vi "Cockpit UDP Receive.vi"(8 "error in":errorcluster, 11 "connection ID":refnum<k16>) -> (0 "error out":errorcluster, 2 "read UDP array":sgl[](array[numeric]), 3 "connection ID out":refnum<k16>)   [LabVIEW 2016]
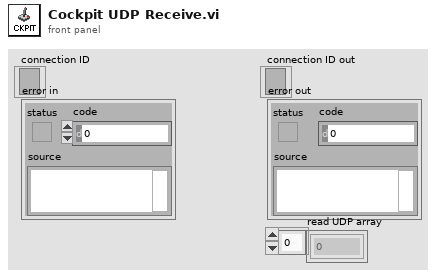
[diagram p1: front panel]
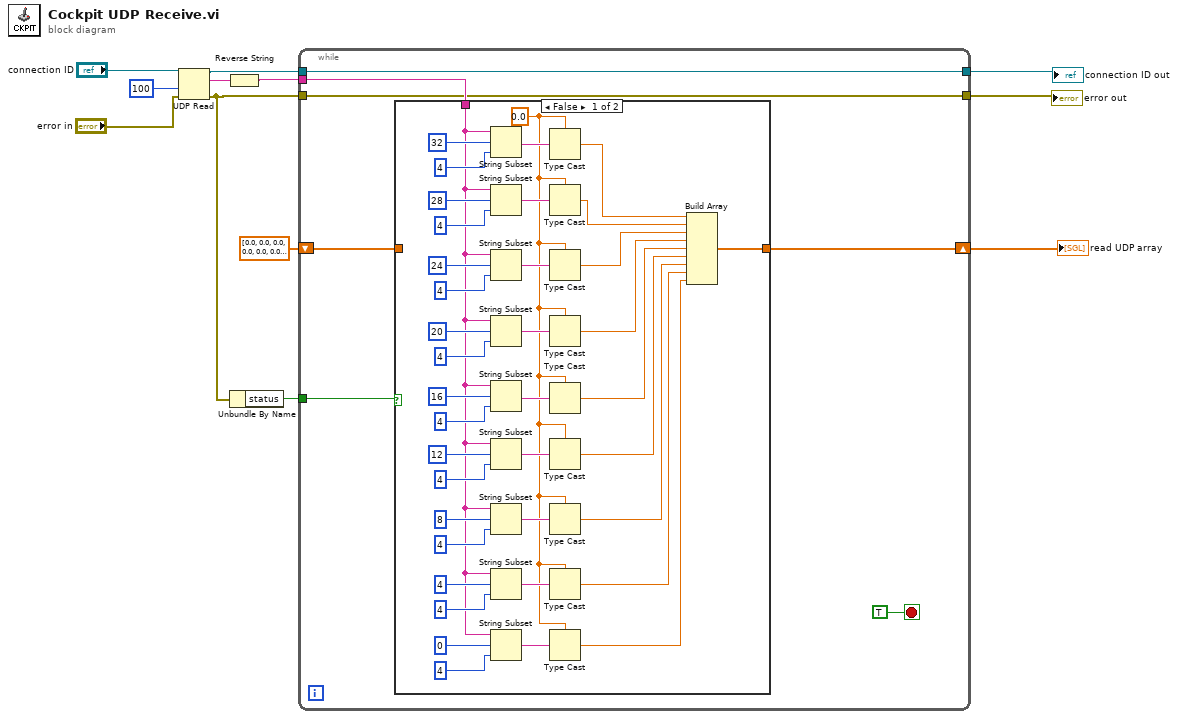
[diagram p0: block diagram]
diagram:
  n1 = UDP Read(connection ID="connection ID", timeout ms (25000)=100, 8:"error in") -> (data out=w8:string, error out=w2:errorcluster, 3:w4:refnum<k16>)  [unwired: 1 in, 2 out]
  n2 = Reverse String(1:w8) -> (0:w7:string)
  n3 = Unbundle By Name(w2) -> ("status"=w3:bool)
  n4 = while {
    tunnel: [w16] -> w12
    tunnel: [w13] -> w11
    shift-right: [w18] -> w10
    shift-left: sgl[] [0.0, 0.0, 0.0, 0.0, 0.0, 0.0, 0.0, 0.0, 0.0] -> [w14]
    tunnel: w7 -> [w17]
    tunnel: w4 -> [w16]
    tunnel: w3 -> [w15]
    tunnel: w2 -> [w13]
    stop <- TRUE stop-if-true
    n5 = case shown="False" w15 {
      tunnel: [w21 w59] -> w18
      tunnel: w17 -> [w20 _]
      tunnel: w14 -> [_ w59]
      frame False {
        w31 = sgl 0.0
        n6 = String Subset(string=w20, offset (0)=32, length (rest)=4 ("offset (0)")) -> (substring=w56:string)
        n7 = String Subset(string=w20, offset (0)=28, length (rest)=4 ("offset (0)")) -> (substring=w49:string)
        n8 = String Subset(string=w20, offset (0)=24, length (rest)=4 ("offset (0)")) -> (substring=w48:string)
        n9 = String Subset(string=w20, offset (0)=20, length (rest)=4 ("offset (0)")) -> (substring=w47:string)
        n10 = String Subset(string=w20, offset (0)=16, length (rest)=4 ("offset (0)")) -> (substring=w38:string)
        n11 = String Subset(string=w20, offset (0)=12, length (rest)=4 ("offset (0)")) -> (substring=w44:string)
        n12 = String Subset(string=w20, offset (0)=8, length (rest)=4 ("offset (0)")) -> (substring=w45:string)
        n13 = String Subset(string=w20, offset (0)=4, length (rest)=4 ("offset (0)")) -> (substring=w46:string)
        n14 = String Subset(string=w20, offset (0)=0, length (rest)=4 ("offset (0)")) -> (substring=w33:string)
        n15 = Type Cast(type=w31, x=w56) -> (*(type *) &x=w30:sgl)
        n16 = Type Cast(type=w31, x=w49) -> (*(type *) &x=w29:sgl)
        n17 = Type Cast(type=w31, x=w48) -> (*(type *) &x=w28:sgl)
        n18 = Type Cast(type=w31, x=w47) -> (*(type *) &x=w27:sgl)
        n19 = Type Cast(type=w31, x=w38) -> (*(type *) &x=w26:sgl)
        n20 = Type Cast(type=w31, x=w44) -> (*(type *) &x=w25:sgl)
        n21 = Type Cast(type=w31, x=w45) -> (*(type *) &x=w24:sgl)
        n22 = Type Cast(type=w31, x=w46) -> (*(type *) &x=w23:sgl)
        n23 = Type Cast(type=w31, x=w33) -> (*(type *) &x=w22:sgl)
        n24 = Build Array(w30, w29, w28, w27, w26, w25, w24, w23, w22) -> (w21:sgl[])
      }
      frame True {
      }
    }
  }
  "connection ID out" <- w12
  "error out" <- w11
  "read UDP array" <- w10
